vi "Sort 2D String Array - Return Format String.vi"(7 "Input String (\" \")":string) -> (8 "Format String":string)   [LabVIEW 2010, in "xijk_select_best_filter.lvlib"]
doc: "Sort 2D String Array - Return Format String.vi\n\n<B>Description:</B>\n\nThis VI finds the meta data (enclosed in <>) in the input string and returns the format string. If the input string does not contain meta data, this VI returns an empty string. \n\n<B>Usage:</B>\n\nWire all required inputs.\n\n<B>Inputs:</B>\n\nInput String\n- The string to scan.\n\n<B>Outputs:</B>\n\nFormat String\n- This is the format string read from the meta data in the input string.\n\n<B>Developed by:</B>\n\nMark Ridgley\nmark.ridgley@logicpd.com"
uses:
  xijk_select_best_filter.lvlib
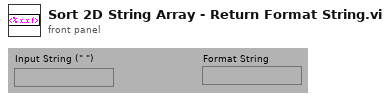
[diagram p1: front panel]
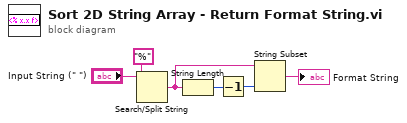
[diagram p0: block diagram]
diagram:
  n1 = Search/Split String(string="Input String (\" \")", search string/char (-)="%" ("search char (-)")) -> (match + rest of string=w3:string)  [unwired: 3 out]
  n2 = String Length(string=w3) -> (length=w5:i32)
  n3 = Decrement(x=w5) -> (x-1=w4:i32)
  n4 = String Subset(string=w3, length (rest)=w4) -> (substring=→"Format String":string)  [unwired: 1 out]
